vi "Step3-2.vi"(1 "d":dbl[][](array[numeric]), 2 "j":i32, 3 "n":i32, 4 "cluster":i32) -> (0 "Array":dbl[][](array[numeric]))   [LabVIEW 2011]
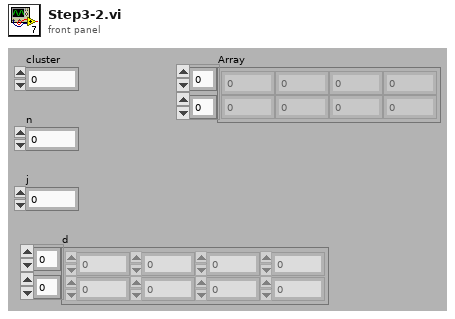
[diagram p1: front panel]
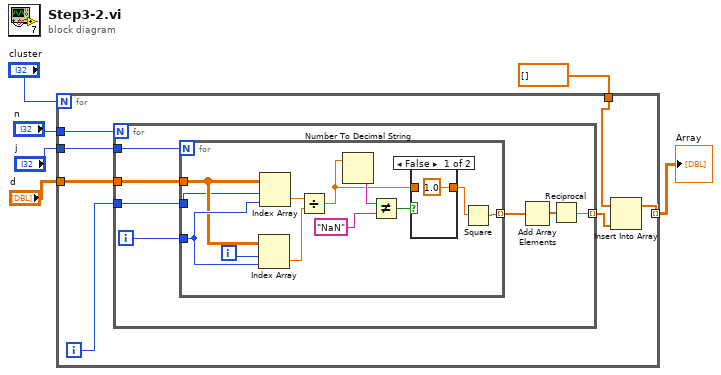
[diagram p0: block diagram]
diagram:
  n1 = for {
    N: "cluster" -> [_]
    tunnel: [w11] -> w1 mode=indexing
    tunnel: dbl[] [] -> [w12]
    tunnel: "n" -> [w9]
    tunnel: "j" -> [w8]
    tunnel: "d" -> [w7]
    i -> [w10]
    n2 = for {
      N: w9 -> [_]
      tunnel: [w18] -> w13 mode=indexing
      tunnel: w10 -> [w16]
      tunnel: w8 -> [w15]
      tunnel: w7 -> [w14]
      i -> [w20]
      n3 = for {
        N: w15 -> [_]
        tunnel: w14 -> [w29]
        tunnel: w20 -> [w32]
        tunnel: [w27] -> w19 mode=indexing
        tunnel: w16 -> [w21]
        i -> [w31]
        n4 = Index Array(array=w29, index (row)=w31, index (col)=w32) -> (element=w28:dbl)
        n5 = Index Array(array=w29, index (row)=w21, index (col)=w32) -> (element=w30:dbl)
        n6 = Divide(x=w30, y=w28) -> (x/y=w22:dbl)
        n7 = Number To Decimal String(number=w22) -> (decimal integer string=w24:string)  [unwired: 1 in]
        n8 = Not Equal?(x=w24, y="NaN") -> (x != y?=w26:bool)
        n9 = case shown="False" w26 {
          tunnel: w22 -> [_ w34]
          tunnel: [1.0 w34] -> w25
          frame False {
          }
          frame True {
          }
        }
        n10 = Square(x=w25) -> (x^2=w27:dbl)
      }
      n11 = Add Array Elements(numeric array=w19) -> (sum=w17:dbl)
      n12 = Reciprocal(x=w17) -> (1/x=w18:dbl)
    }
    n13 = Insert Into Array(array=w12, new element=w13) -> (w11:dbl[])  [unwired: 1 in]
  }
  "Array" <- w1
